vi "MecaKinematics_ToWheelSpeedsZeroCenter.vi"(9 "ChassisSpeeds":T5 {"vOmega" format="%10.3f"; "vY" format="%10.3f"; "vX" format="%10.3f"}, 11 "in MECA_DRIVE_KINEMATICS":T1={"FrontLeft"={"X"=0.0, "Y"=0.0}, "FrontRight"={"X"=0.0, "Y"=0.0}, "RearLeft"={"X"=0.0, "Y"=0.0}, "RearRight"={"X"=0.0, "Y"=0.0}, "InverseKinematics"=[[0.0, 1.0, -1.0, 0.0], [0.0, 1.0, 1.0, 0.0], [0.0, 1.0, 1.0, 0.0], [0.0, 1.0, -1.0, 0.0]], "ForwardKinematics"=[[0.0, 1.0, -1.0, 0.0], [0.0, 1.0, 1.0, 0.0], [0.0, 1.0, 1.0, 0.0], [0.0, 1.0, -1.0, 0.0]], "PrevCoR"={"X"=0.0, "Y"=0.0}} {"PrevCoR"."Y" format="%14.3f"; "PrevCoR"."X" format="%14.3f"; "RearRight"."Y" format="%14.3f"; "RearRight"."X" format="%14.3f"; "RearLeft"."Y" format="%14.3f"; "RearLeft"."X" format="%14.3f"; "FrontRight"."Y" format="%14.3f"; "FrontRight"."X" format="%14.3f"; "FrontLeft"."Y" format="%14.3f"; "FrontLeft"."X" format="%14.3f"}) -> (1 "MECA_WHEEL_SPEEDS":T4 {"RearRightSpeed" format="%19.3f"; "RearLeftSpeed" format="%19.3f"; "FrontRightSpeed" format="%19.3f"; "FrontLeftSpeed" format="%19.3f"}, 3 "out MECA_DRIVE_KINEMATICS":T1={"FrontLeft"={"X"=0.0, "Y"=0.0}, "FrontRight"={"X"=0.0, "Y"=0.0}, "RearLeft"={"X"=0.0, "Y"=0.0}, "RearRight"={"X"=0.0, "Y"=0.0}, "InverseKinematics"=[[0.0, 1.0, -1.0, 0.0], [0.0, 1.0, 1.0, 0.0], [0.0, 1.0, 1.0, 0.0], [0.0, 1.0, -1.0, 0.0]], "ForwardKinematics"=[[0.0, 1.0, -1.0, 0.0], [0.0, 1.0, 1.0, 0.0], [0.0, 1.0, 1.0, 0.0], [0.0, 1.0, -1.0, 0.0]], "PrevCoR"={"X"=0.0, "Y"=0.0}} {"PrevCoR"."Y" format="%14.3f"; "PrevCoR"."X" format="%14.3f"; "RearRight"."Y" format="%14.3f"; "RearRight"."X" format="%14.3f"; "RearLeft"."Y" format="%14.3f"; "RearLeft"."X" format="%14.3f"; "FrontRight"."Y" format="%14.3f"; "FrontRight"."X" format="%14.3f"; "FrontLeft"."Y" format="%14.3f"; "FrontLeft"."X" format="%14.3f"})   [LabVIEW 2019, in "Trajectory_Library.lvlib"]
doc: "Performs inverse kinematics to return the wheel speeds from a desired chassis velocity. This method is often used to convert joystick values into wheel speeds.\n \nDuring normal operations, the center of rotation is usually the same as the physical center of the robot. This subVI, uses the physical center of the robot. Use MecaKinematics_ToWheelSpeeds to use a different center of rotation.\n \nParameters:\n - MecaDriveKinematics - Data structure\n - chassisSpeeds - The desired chassis speed.\n\nReturns:\n - MecaDriveKinematics - Updated data structure\n - WheelSpeeds - The wheel speeds. Use caution because they are not normalized. Sometimes, a user input may cause one of the wheel speeds to go above the attainable max velocity. Use the MecaWheel_normalize function to rectify this issue."
uses:
  Trajectory_Library.lvlib
  TypeDef/TRANSLATION2D.ctl
  TypeDef/CHASSIS_SPEEDS.ctl
  TypeDef/MECA_WHEEL_SPEEDS.ctl
  <vilib>/Analysis/Matrix/Datatypes/RealMatrix.ctl
  <vilib>/Analysis/Matrix/NI_Matrix.lvlib
  TypeDef/MECA_DRIVE_KINEMATICS.ctl
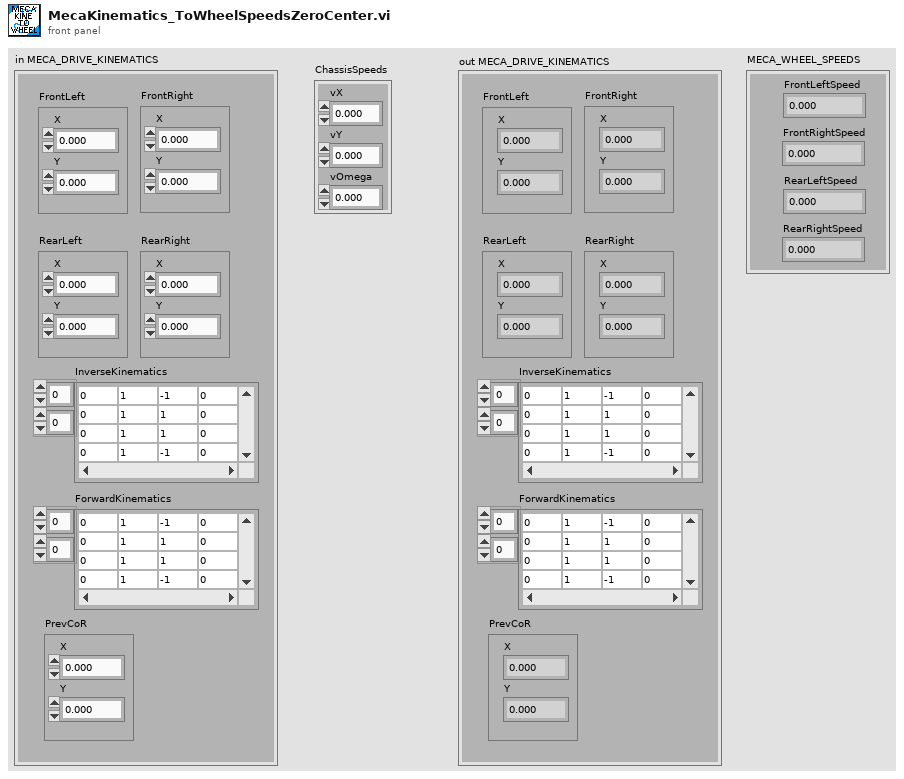
[diagram p1: front panel]
types:
  T1 = typedef "Trajectory_Library.lvlib/MECA_DRIVE_KINEMATICS.ctl" = cluster{"FrontLeft":T2, "FrontRight":T2, "RearLeft":T2, "RearRight":T2, "InverseKinematics":T3, "ForwardKinematics":T3, "PrevCoR":T2}
  T2 = typedef "Trajectory_Library.lvlib/TRANSLATION2D.ctl" = cluster{"X":dbl, "Y":dbl}
  T3 = typedef "NI_Matrix.lvlib/RealMatrix.ctl" = dbl[][]
  T4 = typedef "Trajectory_Library.lvlib/MECA_WHEEL_SPEEDS.ctl" = cluster{"FrontLeftSpeed":dbl, "FrontRightSpeed":dbl, "RearLeftSpeed":dbl, "RearRightSpeed":dbl}
  T5 = typedef "Trajectory_Library.lvlib/CHASSIS_SPEEDS.ctl" = cluster{"vX":dbl, "vY":dbl, "vOmega":dbl}
  T6 = typedef "WPILib_Math.lvlib/TRANSLATION2D.ctl" = cluster{"X":dbl, "Y":dbl}
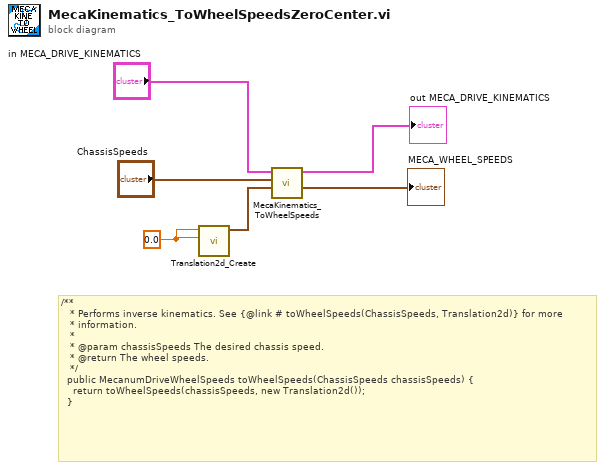
[diagram p0: block diagram]
diagram:
  w2 = 0.0 ("Y")
  # "/**\n   * Performs inverse kinematics. See {@link # toWheelSpeeds(ChassisSpeeds, Translation2d)} for more\n   * information.\n   *\n   * @param chassisSpeeds The desired chassis speed.\n   * @return The wheel speeds.\n   */\n  public MecanumDriveWheelSpeeds toWheelSpeeds(ChassisSpeeds chassisSpeeds) {\n    return toWheelSpeeds(chassisSpeeds, new Translation2d());\n  }"
  n1 = call "Translation2d_Create.vi"("Y"=w2, "X"=w2) -> ("TRANSLATION"=w1:T6)  [unwired: 9 in]
  n2 = call "MecaKinematics_ToWheelSpeeds.vi"("CenterOfRotation"=w1, "ChassisSpeeds"="ChassisSpeeds", "in MECA_DRIVE_KINEMATICS"="in MECA_DRIVE_KINEMATICS") -> ("MECA_WHEEL_SPEEDS"=→"MECA_WHEEL_SPEEDS":T4, "out MECA_DRIVE_KINEMATICS"=→"out MECA_DRIVE_KINEMATICS":T1)  [unwired: 7 in]
